vi "Get User Request.vi"(0 "Serial port assistant view in":refnum<class "Serial port assistant view.lvclass">, 11 "error in (no error)":errorcluster) -> (4 "Serial port assistant view out":refnum<class "Serial port assistant view.lvclass">, 6 "Model Name":string, 8 "Model Number":i32, 10 "Request":string, 15 "error out":errorcluster)   [LabVIEW 2022 SP3, in "Serial port assistant view.lvlib" / "Serial port assistant view.lvclass"]
uses:
  Serial port assistant view.lvclass
  Serial port assistant view.lvclass/Serial port assistant view.ctl
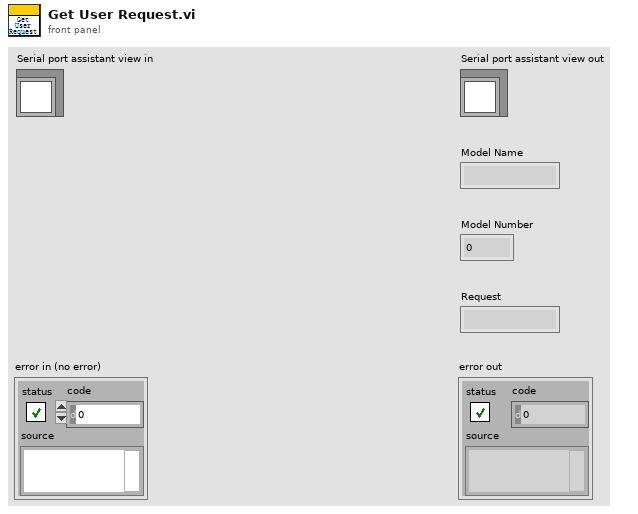
[diagram p1: front panel]
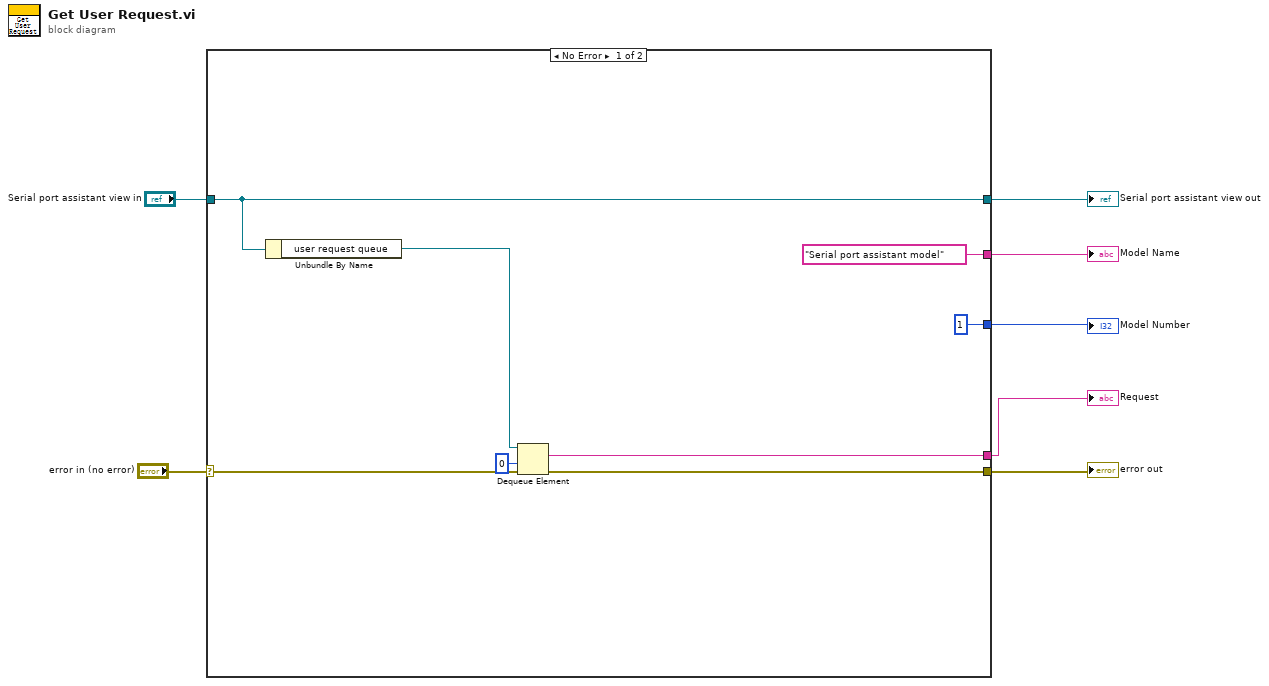
[diagram p0: block diagram]
diagram:
  n1 = case shown="No Error" "error in (no error)" {
    selector: "error in (no error)" -> [w14 w17]
    tunnel: [w13 w17] -> w6
    tunnel: "Serial port assistant view in" -> [w15 w16]
    tunnel: [w15 w16] -> w4
    tunnel: ["Serial port assistant model" _] -> w3
    tunnel: [w11 _] -> w2
    tunnel: [1 ("Model Number") _] -> w1
    frame No Error {
      n2 = Unbundle By Name(w15) -> ("user request queue"=w12:refnum<queue>)
      n3 = Dequeue Element(queue=w12, timeout in ms (-1)=0, error in (no error)=w14) -> (element=w11:string, error out=w13:errorcluster)  [unwired: 2 out]
    }
    frame Error {
    }
  }
  "error out" <- w6
  "Serial port assistant view out" <- w4
  "Model Name" <- w3
  "Request" <- w2
  "Model Number" <- w1
